vi "DFT normalizada.vi"(10 "FFT size":i32, 11 "X":dbl[](array[numeric])) -> (3 "DFT X":dbl[](array[numeric]))   [LabVIEW 2020]
uses:
  <vilib>/Analysis/2dsp.llb/Real FFT.vi
  <vilib>/Analysis/NI_AALPro.lvlib
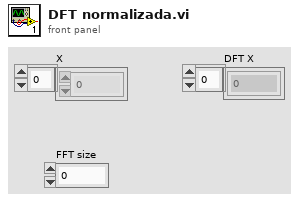
[diagram p1: front panel]
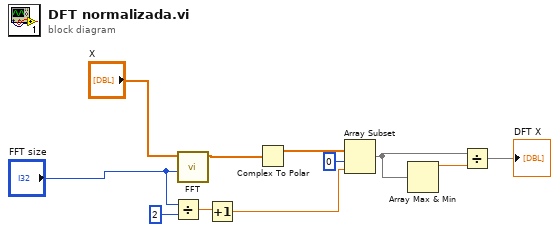
[diagram p0: block diagram]
diagram:
  n1 = Divide(x="FFT size", y=2) -> (x/y=w6:dbl)
  n2 = call-poly <vilib>:"FFT.vi"("FFT size"="FFT size", "X"="X") -> ("FFT {X}"=w8:cdb[])  [unwired: 8 in, 1 out]
  n3 = Increment(x=w6) -> (x+1=w5:dbl)
  n4 = Complex To Polar(r * e^(i*theta)=w8) -> (r=w7:dbl[])  [unwired: 1 out]
  n5 = Array Subset(array=w7, index=0, length=w5) -> (w3:dbl[])
  n6 = Array Max & Min(array=w3) -> (max value=w4:dbl)  [unwired: 3 out]
  n7 = Divide(x=w3, y=w4) -> (x/y=→"DFT X":dbl[])
